vi "Handle.vi"(7 "Queue jettl in":refnum<class "Queue Actor.lvclass">, 11 "Error State in":refnum<class "Error State.lvclass">) -> (2 "Destroy?":bool, 5 "Queue jettl out":refnum<class "Queue Actor.lvclass">)   [LabVIEW 2021, in "jettl.lvlib" / "Base Queue jettl.lvlib" / "Error State.lvclass"]
uses:
  Error State.lvclass
  Actor/Queue Actor/Queue Actor.lvclass
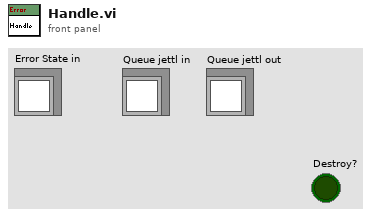
[diagram p1: front panel]
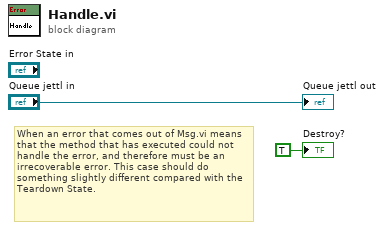
[diagram p0: block diagram]
diagram:
  # "When an error that comes out of Msg.vi means that the method that has executed could not handle the error, and therefore must be an irrecoverable error. This case should do something slightly different compared with the Teardown State."
  "Destroy?" <- TRUE ("Destroy?")
  "Queue jettl out" <- "Queue jettl in"
